vi "first vi.vi"() -> ()   [LabVIEW 2025]
panel:
  out "String":string
  out "e":dbl
  out "c":dbl
  out "d":bool
  in  "b":dbl
  in  "a":dbl
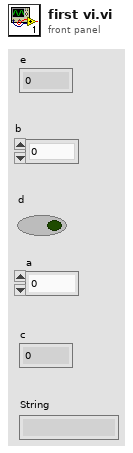
[diagram p1: front panel]
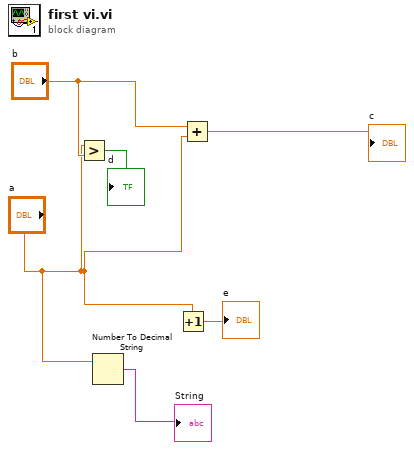
[diagram p0: block diagram]
diagram:
  n1 = Greater?(x="a", y="b") -> (0:→"d":bool)
  n2 = Number To Decimal String(number="a") -> (decimal integer string=→"String":string)  [unwired: 1 in]
  n3 = Increment(x="a") -> (x+1=→"e":dbl)
  n4 = Add(x="b", y="a") -> (x+y=→"c":dbl)
